vi "generate_vector.vi"() -> (0 "Cluster":cluster{"number":dbl, "number":dbl})   [LabVIEW 2023]
uses:
  <vilib>/numeric/Random Number (Range) DBL.vi
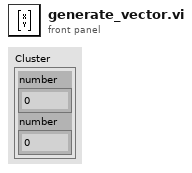
[diagram p1: front panel]
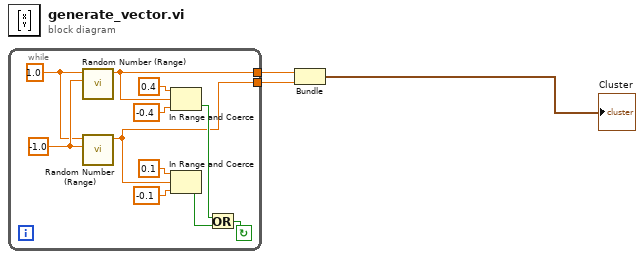
[diagram p0: block diagram]
diagram:
  n1 = while {
    tunnel: [w9] -> w2
    tunnel: [w8] -> w3
    stop <- w10 continue-if-true
    w14 = -1.0 ("lower bound (0)")
    w13 = 1.0 ("upper bound (100)")
    n2 = call-poly <vilib>:"Random Number (Range).vi"("lower bound (0)"=w14, "upper bound (100)"=w13) -> ("number"=w9:dbl)  [unwired: 9 in]
    n3 = call-poly <vilib>:"Random Number (Range).vi"("lower bound (0)"=w14, "upper bound (100)"=w13) -> ("number"=w8:dbl)  [unwired: 9 in]
    n4 = In Range and Coerce(upper limit=0.4, x=w9, lower limit=-0.4 ("upper limit")) -> (In Range?=w12:bool)  [unwired: 1 out]
    n5 = In Range and Coerce(upper limit=0.1, x=w8, lower limit=-0.1) -> (In Range?=w11:bool)  [unwired: 1 out]
    n6 = Or(x=w12, y=w11) -> (x .or. y?=w10:bool)
  }
  n7 = Bundle("number"=w2, "number"=w3) -> (→"Cluster":cluster{"number":dbl, "number":dbl})  [unwired: 1 in]
